vi "Test.vi"() -> ()   [LabVIEW 2011]
panel:
  in  "Multicolumn Listbox":i32(listbox)
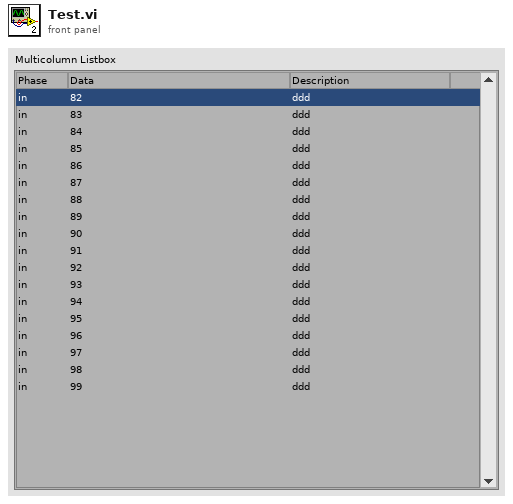
[diagram p1: front panel]
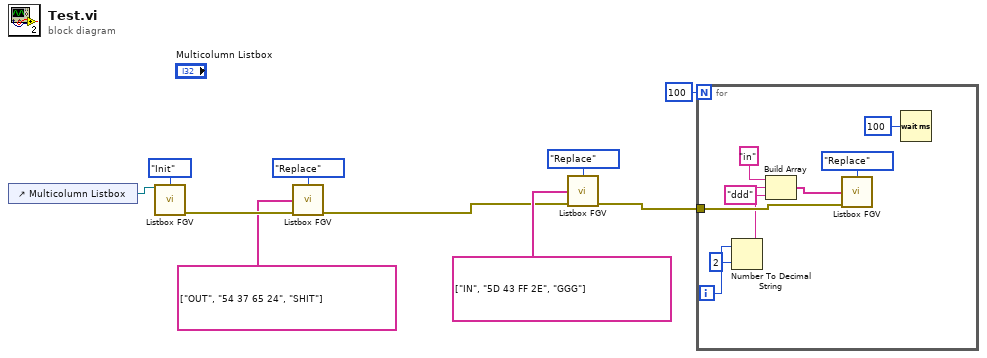
[diagram p0: block diagram]
diagram:
  n1 = control-ref of="Multicolumn Listbox"() -> (w7:refnum<vi>)
  n2 = call "Listbox FGV.vi"("MulticolumnListbox in"=w7, "Enum"=enum16{"Init", "Replace", "Clear"}."Init") -> ("error out"=w8:errorcluster)  [unwired: 12 in, 1 out]
  n3 = call "Listbox FGV.vi"("Enum"=enum16{"Init", "Replace", "Clear"}."Replace", "Array"=string[] ["OUT", "54 37 65 24", "SHIT"], "error in"=w8) -> ("error out"=w3:errorcluster)  [unwired: 11 in, 1 out]
  n4 = call "Listbox FGV.vi"("Enum"=enum16{"Init", "Replace", "Clear"}."Replace", "Array"=string[] ["IN", "5D 43 FF 2E", "GGG"], "error in"=w3) -> ("error out"=w2:errorcluster)  [unwired: 11 in, 1 out]
  n5 = for {
    N: 100 -> [_]
    tunnel: w2 -> [w18]
    i -> [w15]
    n6 = Number To Decimal String(number=w15, width (-)=i16 2) -> (decimal integer string=w13:string)
    n7 = Build Array("in", w13, "ddd" ("element")) -> (w17:string[])
    n8 = call "Listbox FGV.vi"("Enum"=enum16{"Init", "Replace", "Clear"}."Replace", "Array"=w17, "error in"=w18) -> ()  [unwired: 11 in, 2 out]
    n9 = Wait (ms)(milliseconds to wait=u32 100) -> ()  [unwired: 1 out]
  }
